vi "fourAxisData2Cluster.vi"(11 "2D Data Out in":dbl[][](array[numeric])) -> (3 "output cluster":cluster{"z-err data":dbl[], "u_z-data":dbl[]})   [LabVIEW 2017]
panel:
  in  "Cluster":cluster{"z-err data":dbl[], "u_z-data":dbl[]}
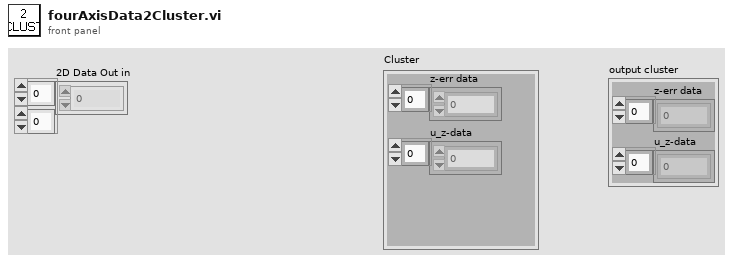
[diagram p1: front panel]
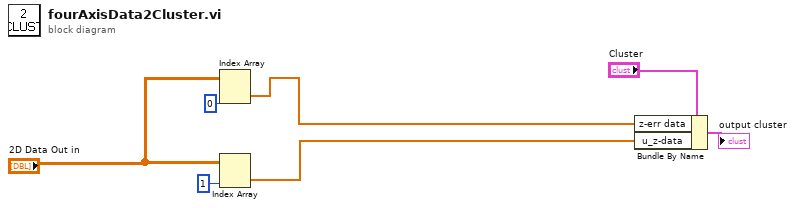
[diagram p0: block diagram]
diagram:
  n1 = Index Array(array="2D Data Out in", index (col)=0) -> (element=w3:dbl[])  [unwired: 1 in]
  n2 = Index Array(array="2D Data Out in", index (col)=1) -> (element=w2:dbl[])  [unwired: 1 in]
  n3 = Bundle By Name(cluster="Cluster", "z-err data"=w3, "u_z-data"=w2) -> (→"output cluster":cluster{"z-err data":dbl[], "u_z-data":dbl[]})
